vi "ReadSubregionLimitsandValue.vi"(0 "object in":refnum<class "Hamamatsu.lvclass">, 5 "error in (no error)":errorcluster) -> (14 "object out":refnum<class "Hamamatsu.lvclass">, 16 "Sub Region":T2 {"V Size"."Value" min=0 max=0 step=4; "H Size"."Value" min=0 max=0 step=4; "V Offset"."Value" min=0 max=0 step=4; "H Offset"."Value" min=0 max=0 step=4}, 19 "error out":errorcluster)   [LabVIEW 2019, in "Hamamatsu.lvclass"]
uses:
  Hamamatsu.lvclass
  <vilib>/Utility/miscctls.llb/LVMinMaxIncTypeDef.ctl
  Hamamatsu.lvclass/Hamamatsu.ctl
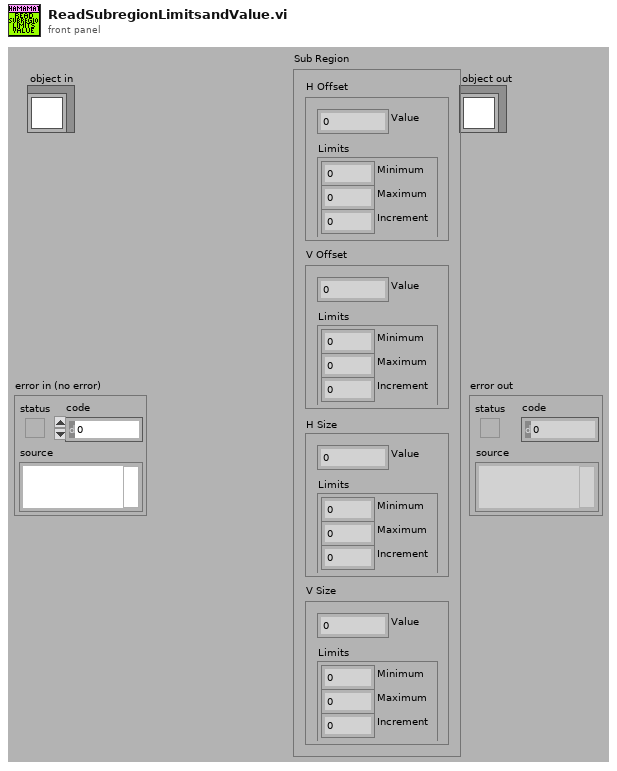
[diagram p1: front panel]
types:
  T1 = typedef "LVMinMaxIncTypeDef.ctl" = cluster{"Minimum":dbl, "Maximum":dbl, "Increment":dbl}
  T2 = cluster{"H Offset":cluster{"Value":i32, "Limits":T1}, "V Offset":cluster{"Value":i32, "Limits":T1}, "H Size":cluster{"Value":i32, "Limits":T1}, "V Size":cluster{"Value":i32, "Limits":T1}}
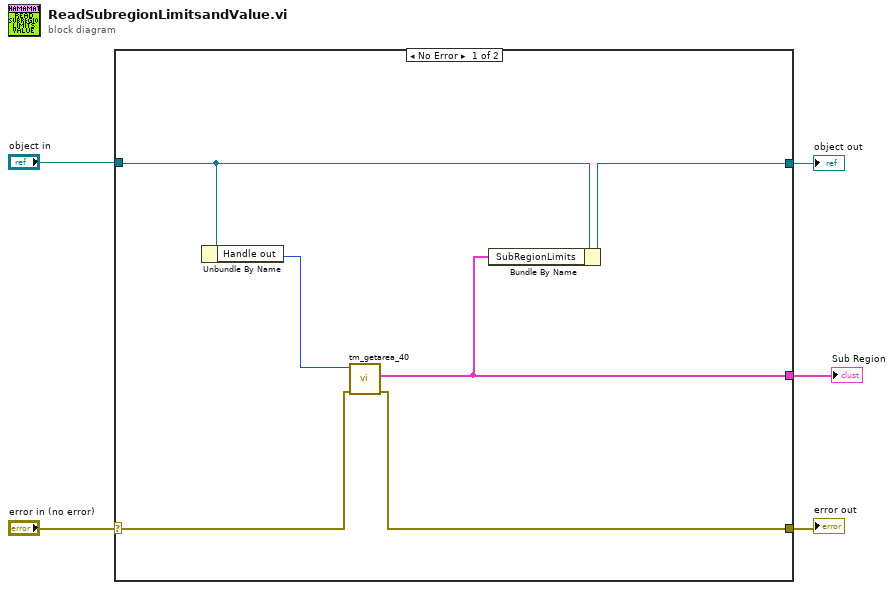
[diagram p0: block diagram]
diagram:
  n1 = case shown="No Error" "error in (no error)" {
    selector: "error in (no error)" -> [w7 w13]
    tunnel: [w6 w13] -> w4
    tunnel: [w10 w12] -> w2
    tunnel: "object in" -> [w11 w12]
    tunnel: [w8 _] -> w1
    frame No Error {
      n2 = Unbundle By Name(w11) -> ("Handle out"=w9:u32)
      n3 = call <userlib>:"tm_getarea_40.vi"("error in (no error)"=w7, "Handle in"=w9) -> ("error out"=w6:errorcluster, "Sub Region"=w8:T2)  [unwired: 7 in, 1 out]
      n4 = Bundle By Name(cluster=w11, "SubRegionLimits"=w8) -> (w10:refnum<class "Hamamatsu.lvclass">)
    }
    frame Error {
    }
  }
  "error out" <- w4
  "object out" <- w2
  "Sub Region" <- w1
